vi "OBST Processing.vi"(1 "OBST":bool, 2 "Line":bool) -> (0 "O/P":bool)   [LabVIEW 2015]
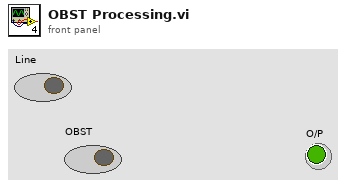
[diagram p1: front panel]
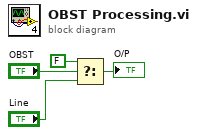
[diagram p0: block diagram]
diagram:
  n1 = Select(t=FALSE, s="OBST", f="Line") -> (s? t:f=→"O/P":bool)
